vi "GetDerivKernels.vi"(6 "normalize":bool, 8 "error in":errorcluster, 9 "kSize":i32=5, 10 "dy":i32=3, 11 "dx":i32=3) -> (0 "error out":errorcluster, 2 "ky":dbl[](array[numeric]), 3 "kx":dbl[](array[numeric]))   [LabVIEW 2020, in "OpenLvVision_OpenCv.lvlib"]
doc: "Returns filter coefficients for computing spatial image derivatives."
uses:
  OpenLvVision_OpenCv.lvlib
  Dlls/OlvOpenCvWrapper.dll
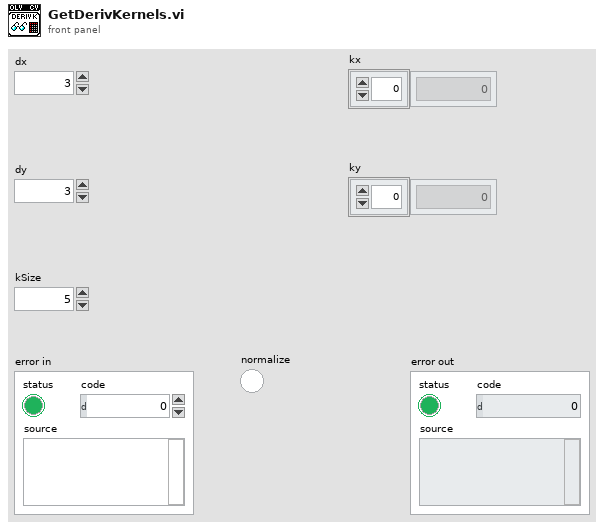
[diagram p1: front panel]
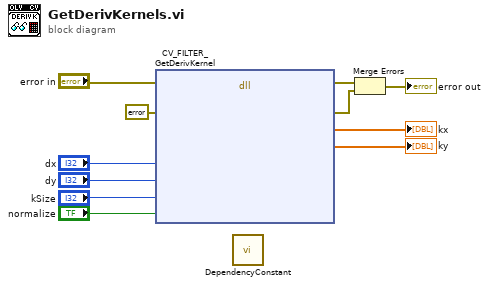
[diagram p0: block diagram]
diagram:
  n1 = dll-call lib="C:/Users/lukas/Downloads/OpenLvVision_OpenCv/SourceCode/LabView/OpenLvVision_OpenCv/Dlls/OlvOpenCvWrapper.dll" fn="CV_FILTER_GetDerivKernel"(error in="error in", "Error"=errorcluster {"status"=FALSE, "code"=0, "source"=""} ("error constant"), "dx"="dx", "dy"="dy", "ksize"="kSize", "normalize"="normalize") -> (error out=w10:errorcluster, "Error"=w9:errorcluster, "kx"=→"kx":dbl[], "ky"=→"ky":dbl[])  [unwired: 9 in, 1 out]
  n2 = call "DependencyConstant.vi"() -> ()  [unwired: 12 in]
  n3 = Merge Errors(w10, w9) -> (→"error out":errorcluster)
